vi "Measure_Select_Current_Range.vi"(1 "Current (A)":dbl) -> (0 "Current Range":i32)   [LabVIEW 2019]
panel:
  out "Current range if this actually worked":i32
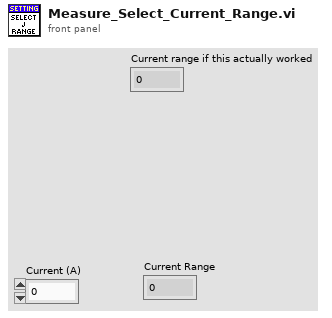
[diagram p1: front panel]
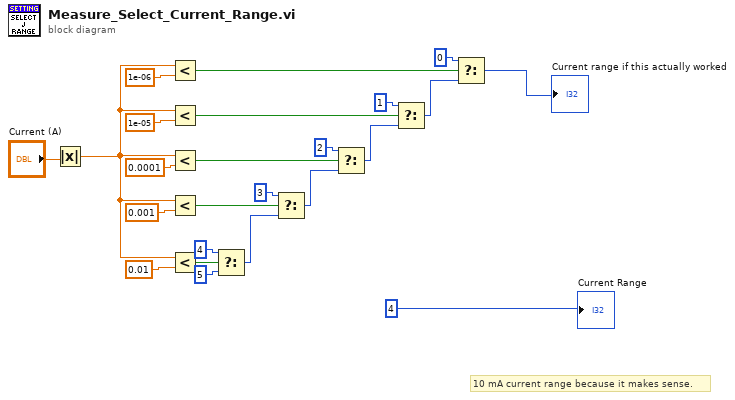
[diagram p0: block diagram]
diagram:
  # "10 mA current range because it makes sense."
  n1 = Absolute Value(x="Current (A)") -> (abs(x)=w2:dbl)
  n2 = Less?(x=w2, y=1e-06) -> (x < y?=w7:bool)
  n3 = Less?(x=w2, y=1e-05) -> (x < y?=w11:bool)
  n4 = Less?(x=w2, y=0.0001) -> (x < y?=w14:bool)
  n5 = Less?(x=w2, y=0.001) -> (x < y?=w21:bool)
  n6 = Less?(x=w2, y=0.01) -> (x < y?=w23:bool)
  n7 = Select(t=4 ("Current Range:\n0=1uA\n1=10uA\n2=100uA\n3=1mA\n4=10mA\n5=120mA"), s=w23, f=5 ("Current Range:\n0=1uA\n1=10uA\n2=100uA\n3=1mA\n4=10mA\n5=120mA")) -> (s? t:f=w19:i32)
  n8 = Select(t=3 ("Current Range:\n0=1uA\n1=10uA\n2=100uA\n3=1mA\n4=10mA\n5=120mA"), s=w21, f=w19) -> (s? t:f=w15:i32)
  n9 = Select(t=2 ("Current Range:\n0=1uA\n1=10uA\n2=100uA\n3=1mA\n4=10mA\n5=120mA"), s=w14, f=w15) -> (s? t:f=w10:i32)
  n10 = Select(t=1 ("Current Range:\n0=1uA\n1=10uA\n2=100uA\n3=1mA\n4=10mA\n5=120mA"), s=w11, f=w10) -> (s? t:f=w8:i32)
  n11 = Select(t=0 ("Current Range:\n0=1uA\n1=10uA\n2=100uA\n3=1mA\n4=10mA\n5=120mA"), s=w7, f=w8) -> (s? t:f=→"Current range if this actually worked":i32)
  "Current Range" <- 4 ("Current Range:\n0=1uA\n1=10uA\n2=100uA\n3=1mA\n4=10mA\n5=120mA")
